vi "Read CSM Doc.vi"(6 "Config Path(\"\" for lvcsm file)":path, 7 "Current Module(\"\" to generate a ID)":string, 8 "error in (no error)":errorcluster, 9 "Force?(F)":bool, 11 "CSM Name":string) -> (0 "Error out":errorcluster, 3 "CSM Doc":string)   [LabVIEW 2020, in "CSM-TCP-Router.lvlib"]
uses:
  CSM-TCP-Router.lvlib
  e8286090-67e2-45e1-b454-2bb1e5cbf17f.vi
  746460eb-3a45-4876-96ec-df97d8415382.vi
  45d20b7d-5e3c-4daf-b7da-62aa04d271f1.vi
  <userlib>/_NEVSTOP/Communicable State Machine(CSM)/AdvanceAPI/CSM - Keywords.vi
  <vilib>/Utility/Data Type/Get Type Information.vi
  <userlib>/_NEVSTOP/Communicable State Machine(CSM)/_csmHelper/lvcsmFile/lvcsm File Path.vi
  <vilib>/Utility/config.llb/Open Config Data.vi
  <vilib>/Utility/config.llb/Write Key.vi
  <vilib>/Utility/config.llb/Write Key (Boolean).vi
  <vilib>/Utility/Data Type/Get Array Information.vi
  <vilib>/Utility/config.llb/Get Key Names.vi
  <vilib>/Utility/config.llb/Remove Key.vi
  <vilib>/Utility/config.llb/Write Key (String).vi
  <userlib>/_NEVSTOP/Communicable State Machine(CSM)/_csmHelper/lvcsmFile/Path to lvcsm String.vi
  <vilib>/Utility/config.llb/Write Key (I32).vi
  <vilib>/Utility/config.llb/Write Key (Double).vi
  <vilib>/Utility/config.llb/Close Config Data.vi
  <vilib>/Utility/config.llb/Read Key.vi
  <vilib>/Utility/config.llb/Read Key (Boolean).vi
  <vilib>/Utility/config.llb/Read Key (String).vi
  <userlib>/_NEVSTOP/Communicable State Machine(CSM)/_csmHelper/lvcsmFile/lvcsm String to Path.vi
  <vilib>/Utility/config.llb/Read Key (I32).vi
  <vilib>/Utility/config.llb/Read Key (Double).vi
  <userlib>/_NEVSTOP/Communicable State Machine(CSM)/_csmHelper/lvcsmFile/_Array of VData to VCluster.vi
  <userlib>/_NEVSTOP/Communicable State Machine(CSM)/Communicable State Machine.lvlib
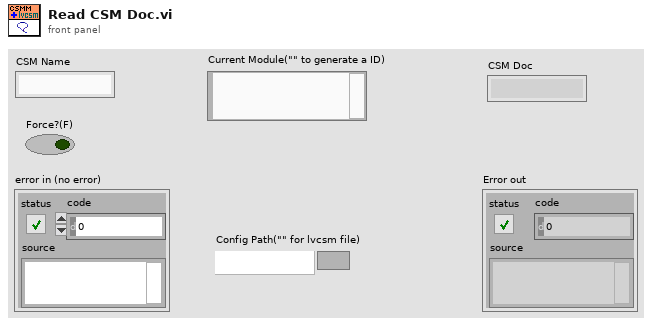
[diagram p1: front panel]
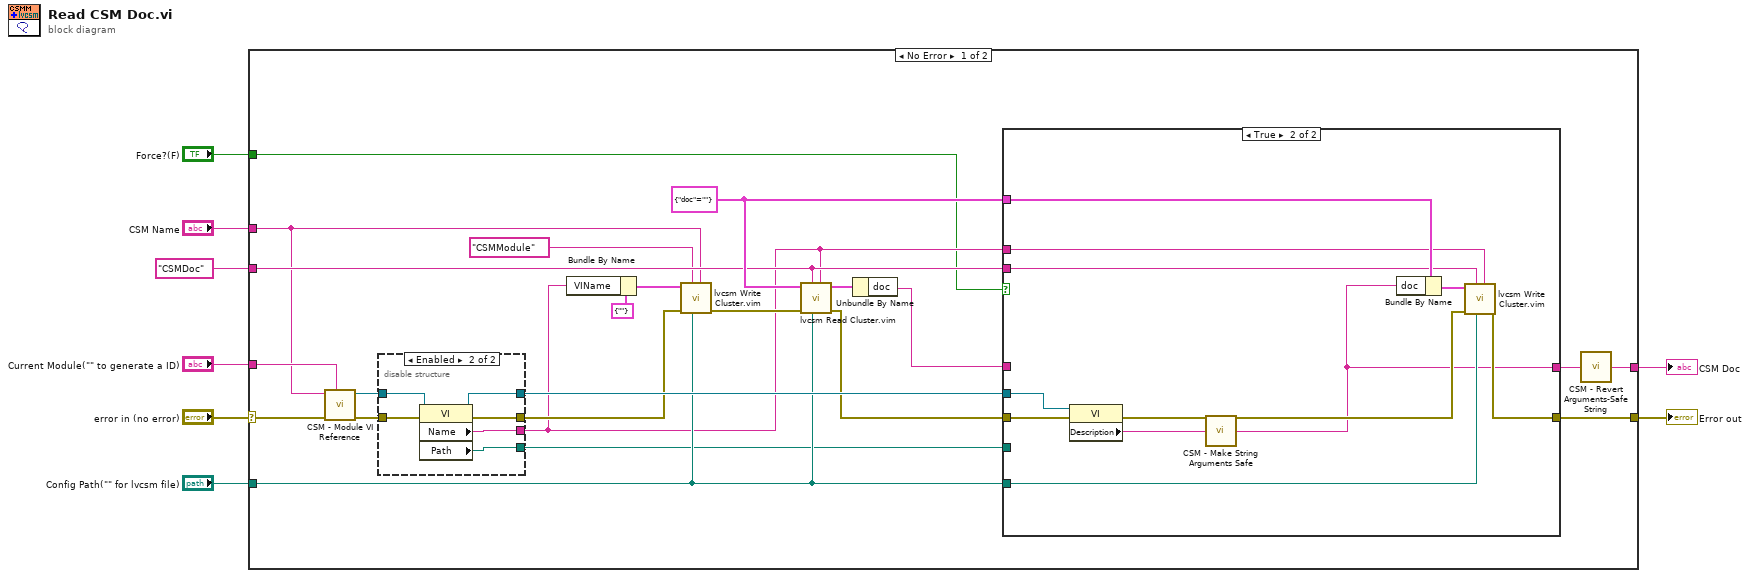
[diagram p0: block diagram]
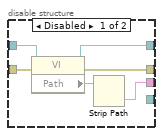
[diagram p2: hidden frame]
diagram:
  n1 = case shown="No Error" "error in (no error)" {
    selector: "error in (no error)" -> [w23 w57]
    tunnel: [w24 w57] -> w3
    tunnel: "CSM Name" -> [w16 _]
    tunnel: "Current Module(\"\" to generate a ID)" -> [w22 _]
    tunnel: [w10 _] -> w2
    tunnel: "Force?(F)" -> [w9 _]
    tunnel: "Config Path(\"\" for lvcsm file)" -> [w19 _]
    tunnel: "CSMDoc" ("API Name") -> [w21 _]
    frame No Error {
      w26 = cluster{"doc":string} {"doc"=""}
      n2 = call <userlib>:"CSM - Module VI Reference.vi"("Current Module (\"\" to Generate an ID)"=w22, "error in (no error)"=w23, "CSM Name"=w16) -> ("error out"=w31:errorcluster, "CSM Module VIRef"=w30:refnum<vi>)  [unwired: 7 in]
      n3 = disable-structure shown="Enabled" {
        disable-tunnel: w31 -> [w37 w43]
        disable-tunnel: w30 -> [w36 w42]
        disable-tunnel: [w35 w41] -> w29
        disable-tunnel: [w33 w40] -> w18
        disable-tunnel: [w32 w39] -> w13
        disable-tunnel: [_ w38] -> w12
        frame Disabled {
          n4 = property class="VI"(reference=w36, error in=w37) -> (reference out=w35:refnum<vi>, error out=w33:errorcluster, "Path"=w34:path)
          n5 = Strip Path(path=w34) -> (name=w32:string)  [unwired: 1 out]
        }
        frame Enabled {
          n6 = property class="VI"(reference=w42, error in=w43) -> (reference out=w41:refnum<vi>, error out=w40:errorcluster, "Name"=w39:string, "Path"=w38:path)
        }
      }
      n7 = Bundle By Name(cluster=cluster{"VIName":string} {"VIName"=""}, "VIName"=w13) -> (w14:cluster{"VIName":string})
      n8 = call "lvcsm Write Cluster.vim"("Sub-section (\"\")"=w16, "Config Path"=w19, "Section"="CSMModule", "Error In"=w18, "Configuration"=w14) -> ("error out"=w20:errorcluster)  [unwired: 6 in]
      n9 = call "lvcsm Read Cluster.vim"("Sub-section (\"\")"=w13, "Config Path"=w19, "Section"=w21, "Error In"=w20, "Default Prototype"=w26) -> ("error out"=w27:errorcluster, "Cluster (Dup)"=w28:cluster{"doc":string})  [unwired: 5 in]
      n10 = Unbundle By Name(w28) -> ("doc"=w25:string)
      n11 = case shown="True" w9 {
        tunnel: w27 -> [w45 w50]
        tunnel: w29 -> [_ w49]
        tunnel: [w45 w54] -> w24
        tunnel: w26 -> [_ w56]
        tunnel: w21 -> [_ w53]
        tunnel: w13 -> [_ w52]
        tunnel: [w44 w46] -> w11
        tunnel: w25 -> [w44 _]
        tunnel: w19 -> [_ w51]
        tunnel: w12 -> [_ _]
        frame False {
        }
        frame True {
          n12 = property class="VI"(reference=w49, error in=w50) -> (error out=w47:errorcluster, "Description"=w48:string)  [unwired: 1 out]
          n13 = call <userlib>:"CSM - Make String Arguments Safe.vi"("Argument String"=w48) -> ("Safe Argument String"=w46:string)  [unwired: 8 in]
          n14 = Bundle By Name(cluster=w56, "doc"=w46) -> (w55:cluster{"doc":string})
          n15 = call "lvcsm Write Cluster.vim"("Sub-section (\"\")"=w52, "Config Path"=w51, "Section"=w53, "Error In"=w47, "Configuration"=w55) -> ("error out"=w54:errorcluster)  [unwired: 6 in]
        }
      }
      n16 = call <userlib>:"CSM - Revert Arguments-Safe String.vi"("Safe Argument String"=w11) -> ("Origin Argument String"=w10:string)  [unwired: 8 in]
    }
    frame Error {
    }
  }
  "Error out" <- w3
  "CSM Doc" <- w2
